vi "NumStringArray (SubVI).vi"(11 "NInt":i32) -> (3 "Array":string[](array[string]))   [LabVIEW 2017, in "LV_Unicorn.lvlib"]
uses:
  LV_Unicorn.lvlib
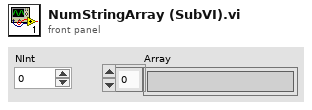
[diagram p1: front panel]
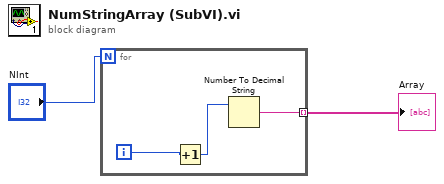
[diagram p0: block diagram]
diagram:
  n1 = for {
    N: "NInt" -> [_]
    tunnel: [w5] -> w2 mode=indexing
    i -> [w4]
    n2 = Increment(x=w4) -> (x+1=w3:i32)
    n3 = Number To Decimal String(number=w3) -> (decimal integer string=w5:string)  [unwired: 1 in]
  }
  "Array" <- w2
